vi "auto sensitivity(SubVI).vi"(8 "error in (no error)":errorcluster, 10 "SR830 num":i32, 11 "config in":T1={"initialize"=enum."SR830", "6221"={"6221 Resource"="GPIB0::24::INSTR", "Delta status"=FALSE, "电流|RMS(A)"=0.0}, "SR830+6221"={"source"=0, "Current(A)"=0.0, "阻抗(Ohm)"=0.0, "SR830 1"=FALSE, "SR830 2"=FALSE, "SR830 3"=FALSE, "SR830 4"=FALSE, "VISA 1"="", "VISA 2"="", "VISA 3"="", "VISA 4"="", "Reserve 1"=0, "Reserve 2"=-1, "Reserve 3"=-1, "Reserve 4"=-1, "Sensitivity 1"=-1, "Sensitivity 2"=0, "Sensitivity 3"=-1, "Sensitivity 4"=-1, "量程入 1"=0, "量程入 2"=0, "量程入 3"=0, "量程入 4"=0}, "2400"={"2400"=FALSE, "VISA"="", "Output Level (0)"=1e-05, "Compliance  Level (0.1)"=10.0}, "ch"={"ch"=[], "current"=[], "change?"=[], "holding current\nwhen change ch?"=FALSE}, "Instrument"={"335 Resource"="GPIB0::24::INSTR", "Input (0:A)"=0, "Instrument Type"=enum."PPMS-Rotate", "quantum design"=refnum, "Heater Output (1:1)"=1, "semaphore"=refnum, "TCP master instance"=refnum, "335 Status"=refnum, "M24C Resource"="GPIB0::24::INSTR", "4G supply"="GPIB0::24::INSTR", "Temp Status 24C"=refnum, "Temp"=refnum, "9T信号"=refnum, "limit"={"Field limit"=0.0, "Field rate limit"=0.0, "Temp limit"=0.0, "Temp low limit"=0.0, "Temp rate limit "=0.0}, "4g supply status"=refnum, "vi路径"="", "325 Resource "="GPIB0::24::INSTR", "Input (0:A) 325"=0, "Input (1;B)"=1, "in-plane"="", "out-plane"="", "in-plane"=FALSE, "out-plane"=FALSE, "in plane 信号"=refnum, "pzt volt"=refnum, "Aborting"=refnum, "数据文件"=refnum, "warning"=refnum, "750 visa"="", "750 rotate"="", "335 Status 2"=refnum}, "2614B"={"2614B chA"=FALSE, "2614B chB"=FALSE, "VISA"=""}, "33522b"={"33522b resource name"="", "零电压"=0.0, "最大电压"=148.0, "间隔"=4.0, "最小电压"=-48.0, "PZT Scan?"=FALSE}, "gating type"=enum."2614(daul)"} {"Instrument"."Input (1;B)" items=["A", "B"]; "Instrument"."Input (0:A) 325" items=["A", "B"]; "Instrument"."Input (0:A)" items=["A", "B"]; "Instrument"."Heater Output (1:1)" items=["1"=1, "2"=2]; "SR830+6221"."Sensitivity 4" items=["Auto Gain"=-1, "2 nV/fA"=0, "5 nV/fA"=1, "10 nV/fA"=2, "20 nV/fA"=3, "50 nV/fA"=4, "100 nV/fA"=5, "200 nV/fA"=6, "500 nV/fA"=7, "1 uV/pA"=8, "2 uV/pA"=9, "5 uV/pA"=10, "10 uV/pA"=11, "20 uV/pA"=12, "50 uV/pA"=13, "100 uV/pA"=14, "200 uV/pA"=15, "500 uV/pA"=16, "1 mV/nA"=17, "2 mV/nA"=18, "5 mV/nA"=19, "10 mV/nA"=20, "20 mV/nA"=21, "50 mV/nA"=22, "100 mV/nA"=23, "200 mV/nA"=24, "500 mV/mA"=25, "1 V/uA"=26]; "SR830+6221"."Sensitivity 3" items=["Auto Gain"=-1, "2 nV/fA"=0, "5 nV/fA"=1, "10 nV/fA"=2, "20 nV/fA"=3, "50 nV/fA"=4, "100 nV/fA"=5, "200 nV/fA"=6, "500 nV/fA"=7, "1 uV/pA"=8, "2 uV/pA"=9, "5 uV/pA"=10, "10 uV/pA"=11, "20 uV/pA"=12, "50 uV/pA"=13, "100 uV/pA"=14, "200 uV/pA"=15, "500 uV/pA"=16, "1 mV/nA"=17, "2 mV/nA"=18, "5 mV/nA"=19, "10 mV/nA"=20, "20 mV/nA"=21, "50 mV/nA"=22, "100 mV/nA"=23, "200 mV/nA"=24, "500 mV/mA"=25, "1 V/uA"=26]; "SR830+6221"."Sensitivity 1" items=["Auto Gain"=-1, "2 nV/fA"=0, "5 nV/fA"=1, "10 nV/fA"=2, "20 nV/fA"=3, "50 nV/fA"=4, "100 nV/fA"=5, "200 nV/fA"=6, "500 nV/fA"=7, "1 uV/pA"=8, "2 uV/pA"=9, "5 uV/pA"=10, "10 uV/pA"=11, "20 uV/pA"=12, "50 uV/pA"=13, "100 uV/pA"=14, "200 uV/pA"=15, "500 uV/pA"=16, "1 mV/nA"=17, "2 mV/nA"=18, "5 mV/nA"=19, "10 mV/nA"=20, "20 mV/nA"=21, "50 mV/nA"=22, "100 mV/nA"=23, "200 mV/nA"=24, "500 mV/mA"=25, "1 V/uA"=26]; "SR830+6221"."Sensitivity 2" items=["Auto Gain"=-1, "2 nV/fA"=0, "5 nV/fA"=1, "10 nV/fA"=2, "20 nV/fA"=3, "50 nV/fA"=4, "100 nV/fA"=5, "200 nV/fA"=6, "500 nV/fA"=7, "1 uV/pA"=8, "2 uV/pA"=9, "5 uV/pA"=10, "10 uV/pA"=11, "20 uV/pA"=12, "50 uV/pA"=13, "100 uV/pA"=14, "200 uV/pA"=15, "500 uV/pA"=16, "1 mV/nA"=17, "2 mV/nA"=18, "5 mV/nA"=19, "10 mV/nA"=20, "20 mV/nA"=21, "50 mV/nA"=22, "100 mV/nA"=23, "200 mV/nA"=24, "500 mV/mA"=25, "1 V/uA"=26]; "SR830+6221"."Reserve 4" items=["Auto Gain"=-1, "2 nV/fA"=0, "5 nV/fA"=1, "10 nV/fA"=2, "20 nV/fA"=3, "50 nV/fA"=4, "100 nV/fA"=5, "200 nV/fA"=6, "500 nV/fA"=7, "1 uV/pA"=8, "2 uV/pA"=9, "5 uV/pA"=10, "10 uV/pA"=11, "20 uV/pA"=12, "50 uV/pA"=13, "100 uV/pA"=14, "200 uV/pA"=15, "500 uV/pA"=16, "1 mV/nA"=17, "2 mV/nA"=18, "5 mV/nA"=19, "10 mV/nA"=20, "20 mV/nA"=21, "50 mV/nA"=22, "100 mV/nA"=23, "200 mV/nA"=24, "500 mV/mA"=25, "1 V/uA"=26]; "SR830+6221"."Reserve 3" items=["Auto Reserve"=-1, "High Reserve"=0, "Normal"=1, "Low Noise"=2]; "SR830+6221"."Reserve 2" items=["Auto Reserve"=-1, "High Reserve"=0, "Normal"=1, "Low Noise"=2]; "SR830+6221"."Reserve 1" items=["Auto Reserve"=-1, "High Reserve"=0, "Normal"=1, "Low Noise"=2]; "SR830+6221"."source" items=["SR830 1", "SR830 2", "SR830 3", "SR830 4"]}) -> (0 "error out":errorcluster, 2 "量程":i32)   [LabVIEW 2019, in "SubVI.lvlib"]
uses:
  SubVI.lvlib
  ctl/config.ctl
  <vilib>/NI/Modbus Library/API/Master/Modbus Master.lvclass
  ctl/initialize.ctl
  ctl/Instrument.ctl
  ctl/Instrument Type.ctl
  lib/QDInstrument.dll
  ctl/335 state.ctl
  ctl/limit.ctl
  ctl/9T mag field stauts.ctl
  ctl/warning.ctl
  ctl/Gating type.ctl
  lib/Stanford Research 830/Stanford Research 830.lvlib
  User lib.lvlib
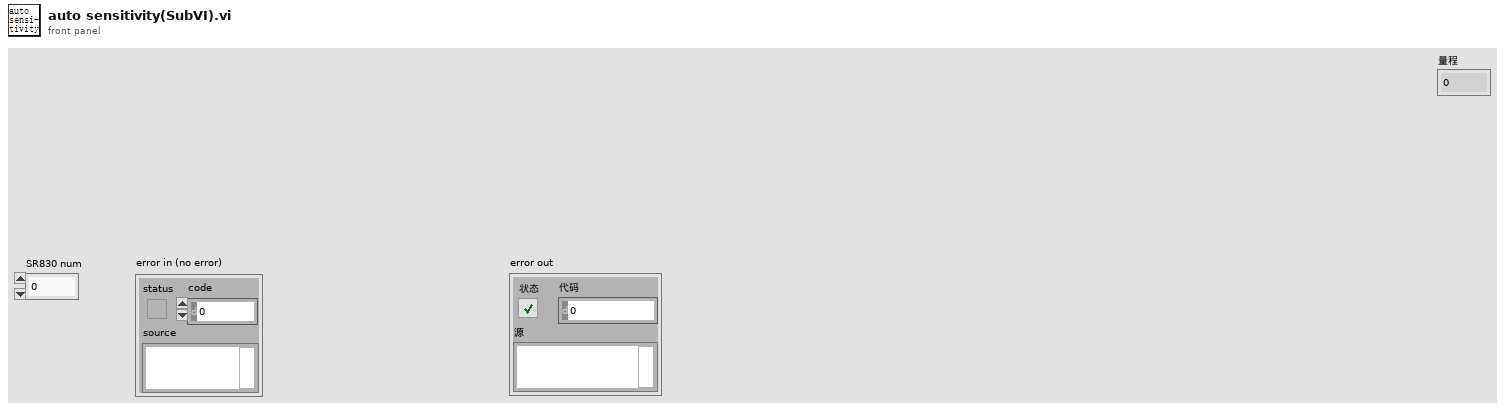
[diagram p1: front panel]
types:
  T1 = typedef "config.ctl" = cluster{"initialize":T2, "6221":cluster{"6221 Resource":refnum<visa-resource-name>, "Delta status":bool, "电流|RMS(A)":dbl}, "SR830+6221":cluster{"source":u16, "Current(A)":dbl, "阻抗(Ohm)":dbl, "SR830 1":bool, "SR830 2":bool, "SR830 3":bool, "SR830 4":bool, "VISA 1":refnum<visa-resource-name>, "VISA 2":refnum<visa-resource-name>, "VISA 3":refnum<visa-resource-name>, "VISA 4":refnum<visa-resource-name>, "Reserve 1":i16, "Reserve 2":i16, "Reserve 3":i16, "Reserve 4":i16, "Sensitivity 1":i16, "Sensitivity 2":i16, "Sensitivity 3":i16, "Sensitivity 4":i16, "量程入 1":i32, "量程入 2":i32, "量程入 3":i32, "量程入 4":i32}, "2400":cluster{"2400":bool, "VISA":refnum<visa-resource-name>, "Output Level (0)":dbl, "Compliance  Level (0.1)":dbl}, "ch":cluster{"ch":i32[], "current":dbl[], "change?":bool[], "holding current\nwhen change ch?":bool}, "Instrument":T3, "2614B":cluster{"2614B chA":bool, "2614B chB":bool, "VISA":refnum<visa-resource-name>}, "33522b":cluster{"33522b resource name":refnum<visa-resource-name>, "零电压":dbl, "最大电压":dbl, "间隔":dbl, "最小电压":dbl, "PZT Scan?":bool}, "gating type":T7}
  T2 = typedef "initialize.ctl" = enum16{"SR830", "keithley6221-SR830", "Delta", "Delta-tunnelling", "keithley6221-2182-DC", "PZT"}
  T3 = typedef "Instrument.ctl" = cluster{"335 Resource":refnum<visa-resource-name>, "Input (0:A)":u16, "Instrument Type":T4, "quantum design":refnum<k24>, "Heater Output (1:1)":u16, "semaphore":T5, "TCP master instance":refnum<class "Modbus Master.lvclass">, "335 Status":refnum<vi>, "M24C Resource":refnum<visa-resource-name>, "4G supply":refnum<visa-resource-name>, "Temp Status 24C":refnum<vi>, "Temp":refnum<vi>, "9T信号":T5, "limit":T6, "4g supply status":refnum<vi>, "vi路径":string, "325 Resource ":refnum<visa-resource-name>, "Input (0:A) 325":u16, "Input (1;B)":u16, "in-plane":refnum<visa-resource-name>, "out-plane":refnum<visa-resource-name>, "in-plane":bool, "out-plane":bool, "in plane 信号":T5, "pzt volt":refnum<vi>, "Aborting":refnum<vi>, "数据文件":refnum<vi>, "warning":refnum<vi>, "750 visa":refnum<visa-resource-name>, "750 rotate":refnum<visa-resource-name>, "335 Status 2":refnum<vi>}
  T4 = typedef "Instrument Type.ctl" = enum16{"PPMS", "VersaLab", "DynaCool", "SVSM", "PPMS-Rotate", "Lakeshore335", "lengtou2", "9T mag", "9T cmag rotate", "test"}
  T5 = typedef "Semaphore RefNum" = refnum<k1>
  T6 = typedef "limit.ctl" = cluster{"Field limit":dbl, "Field rate limit":dbl, "Temp limit":dbl, "Temp low limit":dbl, "Temp rate limit ":dbl}
  T7 = typedef "Gating type.ctl" = enum32{"null", "2614(daul)", "2400"}
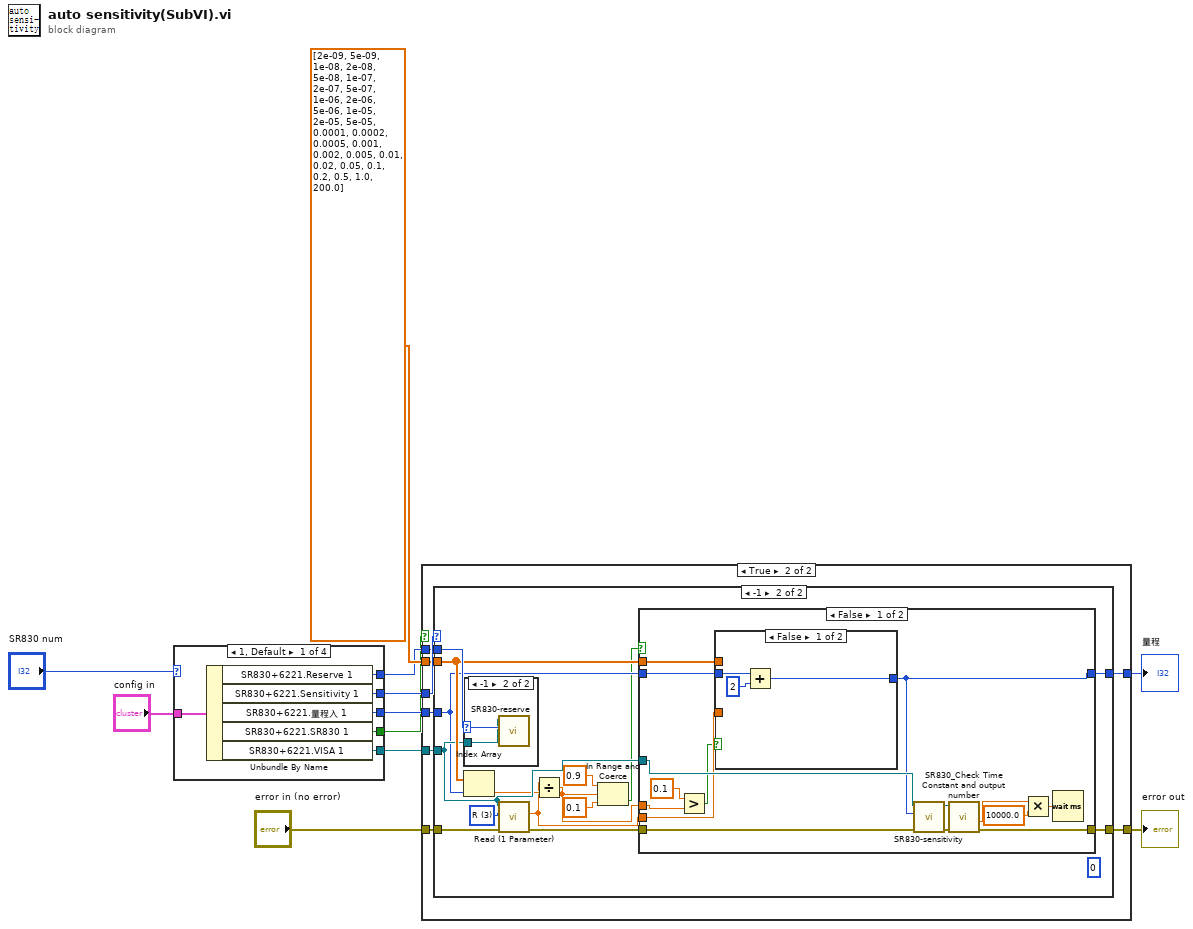
[diagram p0: block diagram]
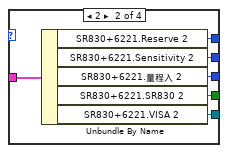
[diagram p2: hidden frame]
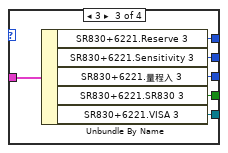
[diagram p3: hidden frame]
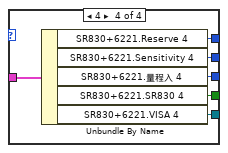
[diagram p4: hidden frame]
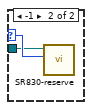
[diagram p7: hidden frame]
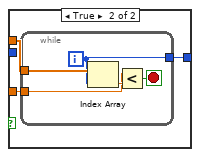
[diagram p8: hidden frame]
diagram:
  n1 = case shown="1, Default" "SR830 num" {
    tunnel: "config in" -> [w17 w23 w29 w35]
    tunnel: [w16 w22 w28 w34] -> w8
    tunnel: [w15 w21 w27 w33] -> w7
    tunnel: [w14 w20 w26 w32] -> w6
    tunnel: [w13 w19 w25 w31] -> w5
    tunnel: [w12 w18 w24 w30] -> w4
    frame 1, Default {
      n2 = Unbundle By Name(w17) -> ("SR830+6221.Reserve 1"=w16:i16, "SR830+6221.Sensitivity 1"=w15:i16, "SR830+6221.量程入 1"=w14:i32, "SR830+6221.SR830 1"=w13:bool, "SR830+6221.VISA 1"=w12:refnum<visa-resource-name>)
    }
    frame 2 {
      n3 = Unbundle By Name(w23) -> ("SR830+6221.Reserve 2"=w22:i16, "SR830+6221.Sensitivity 2"=w21:i16, "SR830+6221.量程入 2"=w20:i32, "SR830+6221.SR830 2"=w19:bool, "SR830+6221.VISA 2"=w18:refnum<visa-resource-name>)
    }
    frame 3 {
      n4 = Unbundle By Name(w29) -> ("SR830+6221.Reserve 3"=w28:i16, "SR830+6221.Sensitivity 3"=w27:i16, "SR830+6221.量程入 3"=w26:i32, "SR830+6221.SR830 3"=w25:bool, "SR830+6221.VISA 3"=w24:refnum<visa-resource-name>)
    }
    frame 4 {
      n5 = Unbundle By Name(w35) -> ("SR830+6221.Reserve 4"=w34:i16, "SR830+6221.Sensitivity 4"=w33:i16, "SR830+6221.量程入 4"=w32:i32, "SR830+6221.SR830 4"=w31:bool, "SR830+6221.VISA 4"=w30:refnum<visa-resource-name>)
    }
  }
  n6 = case shown="True" w5 {
    tunnel: w7 -> [_ w45]
    tunnel: w8 -> [_ w44]
    tunnel: w4 -> [_ w43]
    tunnel: dbl[] [2e-09, 5e-09, 1e-08, 2e-08, 5e-08, 1e-07, 2e-07, 5e-07, 1e-06, 2e-06, 5e-06, 1e-05, 2e-05, 5e-05, 0.0001, 0.0002, 0.0005, 0.001, 0.002, 0.005, 0.01, 0.02, 0.05, 0.1, 0.2, 0.5, 1.0, 200.0] -> [_ w42]
    tunnel: w6 -> [w37 w41]
    tunnel: [w36 w40] -> w10
    tunnel: "error in (no error)" -> [w36 w39]
    tunnel: [w37 w38] -> w1
    frame False {
    }
    frame True {
      n7 = case shown="-1" w45 {
        tunnel: w44 -> [w49 w66]
        tunnel: w43 -> [w48 w64]
        tunnel: w42 -> [_ w65]
        tunnel: w41 -> [w46 w63]
        tunnel: [w47 w54] -> w40
        tunnel: w39 -> [w47 w53]
        tunnel: [w46 w52] -> w38
        frame 0, Default {
          n8 = case shown="0, Default" w49 {
            selector: w49 -> [_ w51]
            tunnel: w48 -> [_ w50]
            frame 0, Default {
            }
            frame -1 {
              n9 = call "SR830-reserve.vi"("Dynamic Reserve (-1: Auto Reserve)"=w51, "VISA resource name"=w50) -> ()  [unwired: 8 in, 2 out]
            }
          }
        }
        frame -1 {
          w62 = u16 3 items=["X"=1, "Y"=2, "R"=3, "Theta"=4, "Channel 1"=5, "Channel 2"=6, "Aux In 1"=7, "Aux In 2"=8, "Aux In 3"=9, "Aux In 4"=10] ("Parameter (1: X)")
          (unwired) 0
          n10 = case shown="-1" w66 {
            selector: w66 -> [_ w96]
            tunnel: w64 -> [_ w95]
            frame 0, Default {
            }
            frame -1 {
              n11 = call "SR830-reserve.vi"("Dynamic Reserve (-1: Auto Reserve)"=w96, "VISA resource name"=w95) -> ()  [unwired: 8 in, 2 out]
            }
          }
          n12 = Index Array(array=w65, index=w63) -> (element=w61:dbl)
          n13 = call "Read (1 Parameter).vi"("error in (no error)"=w53, "Parameter (1: X)"=w62, "VISA resource name"=w64) -> ("error out"=w56:errorcluster, "Measurement"=w57:dbl)  [unwired: 6 in, 1 out]
          n14 = Divide(x=w57, y=w61) -> (x/y=w55:dbl)
          n15 = In Range and Coerce(upper limit=0.9 ("上限"), x=w55, lower limit=0.1 ("下限")) -> (In Range?=w58:bool)  [unwired: 1 out]
          n16 = case shown="False" w58 {
            tunnel: w64 -> [w81 _]
            tunnel: w65 -> [w80 _]
            tunnel: w57 -> [w79 _]
            tunnel: w56 -> [w78 w93]
            tunnel: w55 -> [w76 _]
            tunnel: w63 -> [w77 w94]
            tunnel: [w68 w94] -> w52
            tunnel: [w67 w93] -> w54
            frame False {
              n17 = Greater?(x=0.1 ("y"), y=w76) -> (0:w69:bool)
              n18 = case shown="False" w69 {
                tunnel: w79 -> [_ w87]
                tunnel: [w82 w86] -> w68
                tunnel: w80 -> [_ w85]
                tunnel: w77 -> [w84 _]
                frame False {
                  n19 = Add(x=w84, y=2) -> (x+y=w82:i32)
                }
                frame True {
                  n20 = while {
                    tunnel: w85 -> [w90]
                    tunnel: w87 -> [w89]
                    tunnel: [w88] -> w86
                    i -> [w88]
                    stop <- w92 stop-if-true
                    n21 = Index Array(array=w90, index=w88) -> (element=w91:dbl)
                    n22 = Less?(x=w89, y=w91) -> (x < y?=w92:bool)
                  }
                }
              }
              n23 = call "SR830-sensitivity.vi"("error in (no error)"=w78, "Sensitivity (-1: Auto gain)"=w68, "VISA resource name"=w81) -> ("error out"=w71:errorcluster, "VISA resource name out"=w75:refnum<visa-resource-name>)  [unwired: 7 in]
              n24 = call "SR830_Check Time Constant and output number.vi"("error in (no error)"=w71, "SR830 resource name"=w75) -> ("error out"=w67:errorcluster, "TIme Constant Num"=w74:dbl)  [unwired: 6 in, 2 out]
              n25 = Multiply(x=w74, y=10000.0) -> (x*y=w72:dbl)
              n26 = Wait (ms)(milliseconds to wait=w72) -> ()  [unwired: 1 out]
            }
            frame True {
            }
          }
        }
      }
    }
  }
  "error out" <- w10
  "量程" <- w1
